vi "zone indicators.vi"(8 "error in (no error)":errorcluster, 9 "Time":dbl, 10 "Direction":string, 11 "sprinkler data in":T1) -> (0 "error out":errorcluster, 3 "sprinkler data out":T1)   [LabVIEW 2015]
uses:
  controls/sprinkler data.ctl
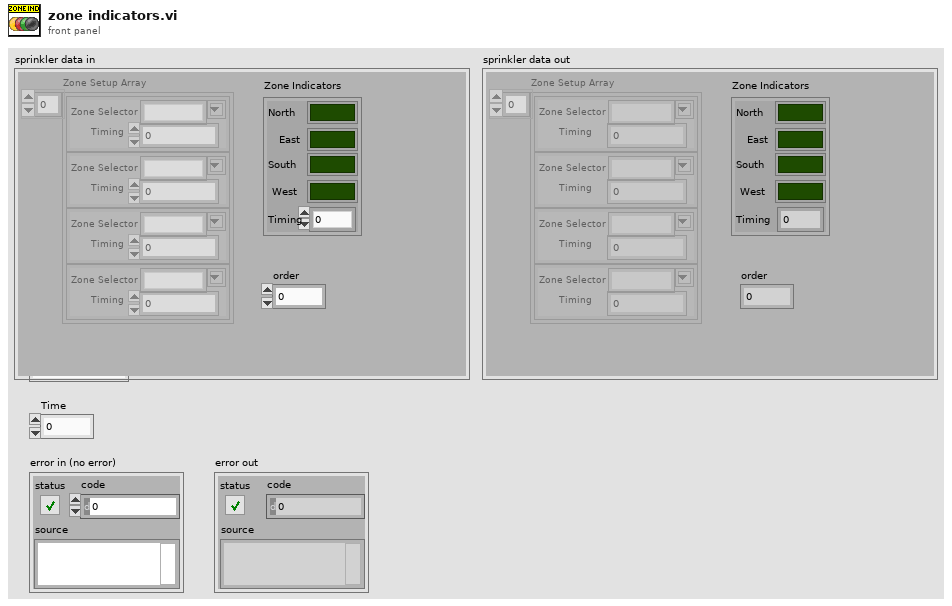
[diagram p1: front panel]
types:
  T1 = typedef "sprinkler data.ctl" = cluster{"Zone Setup Array":cluster{"Zone Selector":string, "Timing":dbl}[], "Zone Indicators":cluster{"North":bool, "East":bool, "South":bool, "West":bool, "Timing":u32}, "order":i32}
  T2 = cluster{"North":bool, "East":bool, "South":bool, "West":bool, "Timing":u32}
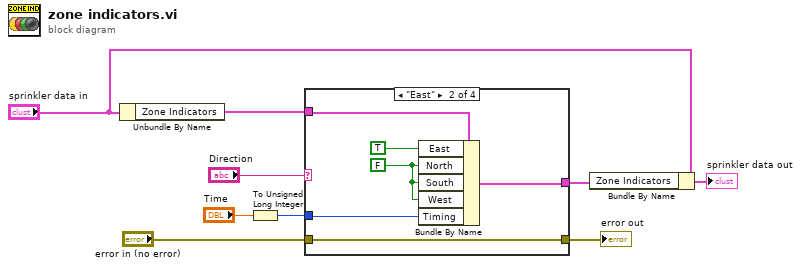
[diagram p0: block diagram]
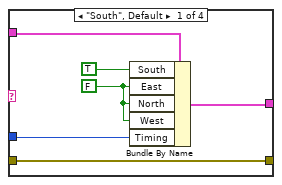
[diagram p2: hidden frame]
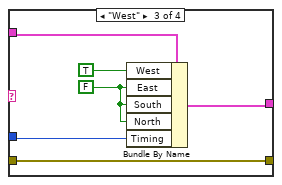
[diagram p3: hidden frame]
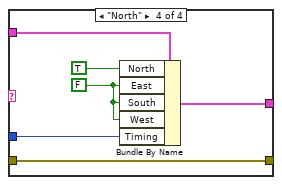
[diagram p4: hidden frame]
diagram:
  n1 = Unbundle By Name("sprinkler data in") -> ("Zone Indicators"=w4:T2)
  n2 = To Unsigned Long Integer(number="Time") -> (unsigned 32bit integer=w7:u32)
  n3 = case shown="\"East\"" "Direction" {
    tunnel: w4 -> [w12 w18 w24 w33]
    tunnel: w7 -> [w13 w19 w25 w32]
    tunnel: [w11 w17 w23 w29] -> w2
    tunnel: "error in (no error)" -> [w10 w16 w22 w28]
    tunnel: [w10 w16 w22 w28] -> w9
    frame "South", Default {
      w14 = FALSE ("East")
      n4 = Bundle By Name(cluster=w12, "South"=TRUE ("North"), "East"=w14, "North"=w14, "West"=w14, "Timing"=w13) -> (w11:T2)
    }
    frame "East" {
      w21 = FALSE ("East")
      n5 = Bundle By Name(cluster=w18, "East"=TRUE ("North"), "North"=w21, "South"=w21, "West"=w21, "Timing"=w19) -> (w17:T2)
    }
    frame "West" {
      w26 = FALSE ("East")
      n6 = Bundle By Name(cluster=w24, "West"=TRUE ("North"), "East"=w26, "South"=w26, "North"=w26, "Timing"=w25) -> (w23:T2)
    }
    frame "North" {
      w30 = FALSE ("East")
      n7 = Bundle By Name(cluster=w33, "North"=TRUE, "East"=w30, "South"=w30, "West"=w30, "Timing"=w32) -> (w29:T2)
    }
  }
  "error out" <- w9
  n8 = Bundle By Name(cluster="sprinkler data in", "Zone Indicators"=w2) -> (→"sprinkler data out":T1)
